vi "Update Digital Pattern Pattern Controls.vi"(8 "error in (no error)":errorcluster, 11 "Page Data in":T1={"SysExp Event"=refnum, "Init done"=FALSE, "Node Ptr"=18446744073709551615, "Ctrl Refs"={"Header"=refnum, "Pattern Plot"=refnum, "Zoom"=refnum, "Select Pattern"=refnum, "Add List"=refnum, "Remove List"=refnum, "Pattern Name"=refnum, "remove_add"=refnum, "remove_remove"=refnum, "add_remove"=refnum, "base_Length"=refnum, "base_teeth"=refnum, "base_Toothwidth"=refnum, "base_Offset"=refnum, "add_Tooth"=refnum, "add_Width"=refnum, "add_Offset"=refnum, "remove_Tooth"=refnum, "remove_Edge"=refnum, "Chart_Position"=refnum, "Chart_Tooth"=refnum, "Chart_Offset"=refnum, "add_add"=refnum, "pattern_remove"=refnum, "pattern_add"=refnum, "FPGA Resource"=refnum}, "SE ref"=refnum, "Patterns"=[], "Sel patterns"=[], "rotations"=0, "Need save"=FALSE, "Rem List"=0, "Add List"=0, "FPGA Resources"=[]} {"Node Ptr" format="%.0x"}) -> (0 "error out":errorcluster)   [LabVIEW 2017, in "Engine Simulation Toolkit System Explorer.lvlib"]
uses:
  Engine Simulation Toolkit System Explorer.lvlib
  Digital Patterns Page Data.ctl
  <vilib>/NI Veristand/Custom Device API/Custom Device Item Ref.ctl
  Digital Pattern.ctl
  Digital Pattern Base.ctl
  Digital Pattern Remove Edge.ctl
  Digital Pattern Add Pulse.ctl
  <vilib>/NI Veristand/Custom Device API/Custom Device API.lvlib
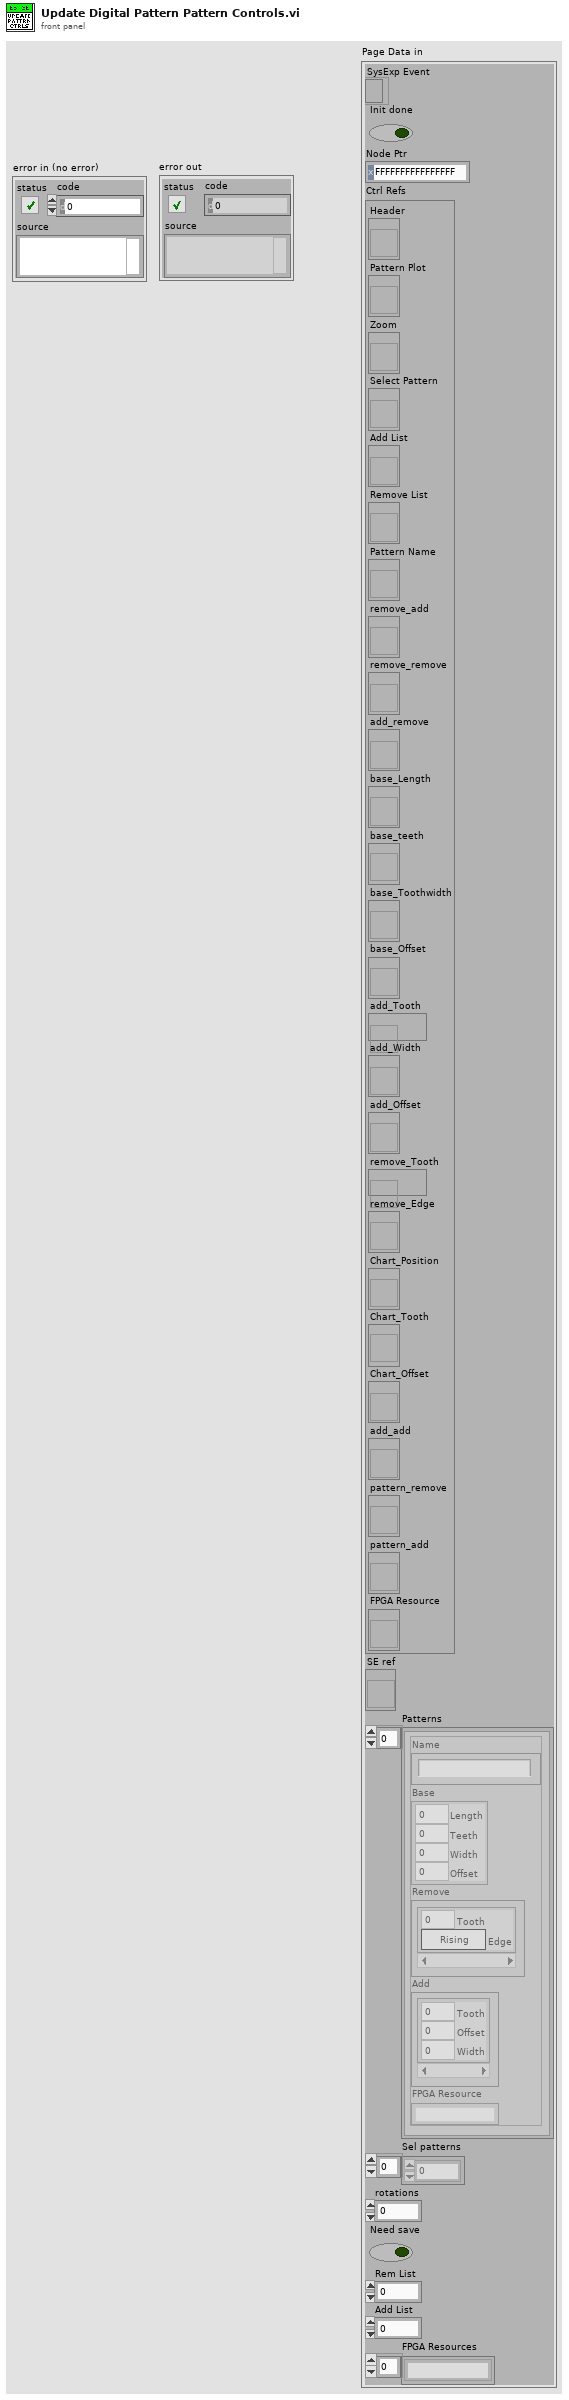
[diagram p1: front panel]
types:
  T1 = typedef "Engine Simulation Toolkit System Explorer.lvlib/Digital Patterns Page Data.ctl" = cluster{"SysExp Event":refnum<event-registration>, "Init done":bool, "Node Ptr":T2, "Ctrl Refs":cluster{"Header":refnum<vi>, "Pattern Plot":refnum<vi>, "Zoom":refnum<vi>, "Select Pattern":refnum<vi>, "Add List":refnum<vi>, "Remove List":refnum<vi>, "Pattern Name":refnum<vi>, "remove_add":refnum<vi>, "remove_remove":refnum<vi>, "add_remove":refnum<vi>, "base_Length":refnum<vi>, "base_teeth":refnum<vi>, "base_Toothwidth":refnum<vi>, "base_Offset":refnum<vi>, "add_Tooth":refnum<vi>, "add_Width":refnum<vi>, "add_Offset":refnum<vi>, "remove_Tooth":refnum<vi>, "remove_Edge":refnum<vi>, "Chart_Position":refnum<vi>, "Chart_Tooth":refnum<vi>, "Chart_Offset":refnum<vi>, "add_add":refnum<vi>, "pattern_remove":refnum<vi>, "pattern_add":refnum<vi>, "FPGA Resource":refnum<vi>}, "SE ref":refnum<vi>, "Patterns":T3[], "Sel patterns":i32[], "rotations":u16, "Need save":bool, "Rem List":i32, "Add List":i32, "FPGA Resources":string[]}
  T2 = typedef "Custom Device API.lvlib/Custom Device Item Ref.ctl" = u64
  T3 = typedef "Engine Simulation Toolkit System Explorer.lvlib/Digital Pattern.ctl" = cluster{"Name":string, "Base":T4, "Remove":T5[], "Add":T6[], "FPGA Resource":string}
  T4 = typedef "Engine Simulation Toolkit System Explorer.lvlib/Digital Pattern Base.ctl" = cluster{"Length":dbl, "Teeth":u16, "Width":dbl, "Offset":dbl}
  T5 = typedef "Engine Simulation Toolkit System Explorer.lvlib/Digital Pattern Remove Edge.ctl" = cluster{"Tooth":u16, "Edge":bool}
  T6 = typedef "Engine Simulation Toolkit System Explorer.lvlib/Digital Pattern Add Pulse.ctl" = cluster{"Tooth":u16, "Offset":dbl, "Width":dbl}
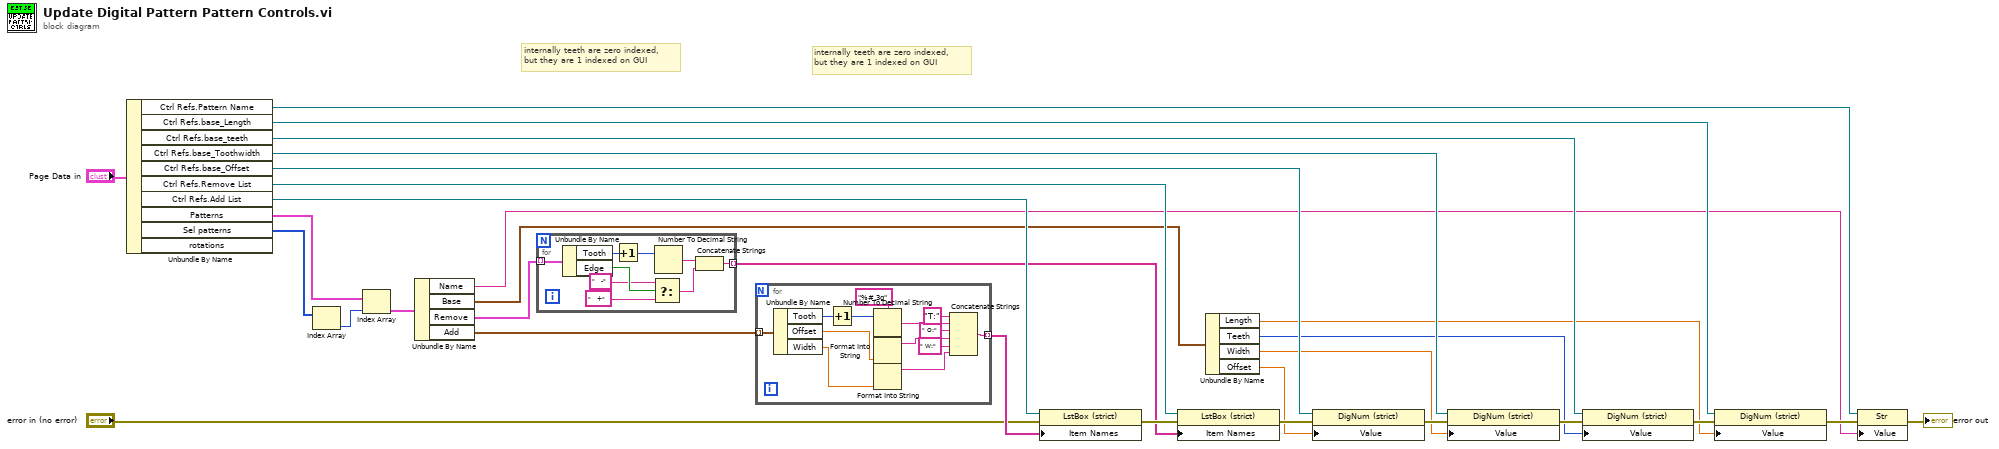
[diagram p0: block diagram]
diagram:
  # "internally teeth are zero indexed, but they are 1 indexed on GUI"
  # "internally teeth are zero indexed, but they are 1 indexed on GUI"
  n1 = Unbundle By Name("Page Data in") -> ("Ctrl Refs.Pattern Name"=w7:refnum<vi>, "Ctrl Refs.base_Length"=w10:refnum<vi>, "Ctrl Refs.base_teeth"=w12:refnum<vi>, "Ctrl Refs.base_Toothwidth"=w15:refnum<vi>, "Ctrl Refs.base_Offset"=w17:refnum<vi>, "Ctrl Refs.Remove List"=w20:refnum<vi>, "Ctrl Refs.Add List"=w24:refnum<vi>, "Patterns"=w2:T3[], "Sel patterns"=w29:i32[])  [unwired: 1 out]
  n2 = Index Array(array=w29) -> (element=w28:i32)  [unwired: 1 in]
  n3 = Index Array(array=w2, index=w28) -> (element=w27:T3)
  n4 = Unbundle By Name(w27) -> ("Name"=w6:string, "Base"=w19:T4, "Remove"=w23:T5[], "Add"=w26:T6[])
  n5 = for {
    tunnel: w23 -> [w39] mode=indexing
    tunnel: [w32] -> w21 mode=indexing
    n6 = Unbundle By Name(w39) -> ("Tooth"=w38:u16, "Edge"=w36:bool)
    n7 = Increment(x=w38) -> (x+1=w31:u16)
    n8 = Select(t="   -" ("string"), s=w36, f="   +" ("string")) -> (s? t:f=w35:string)
    n9 = Number To Decimal String(number=w31) -> (decimal integer string=w37:string)  [unwired: 1 in]
    n10 = Concatenate Strings(w37, w35) -> (w32:string)
  }
  n11 = for {
    tunnel: w26 -> [w52] mode=indexing
    tunnel: [w49] -> w25 mode=indexing
    w42 = "%#.3g" ("format string")
    n12 = Unbundle By Name(w52) -> ("Tooth"=w51:u16, "Offset"=w46:dbl, "Width"=w45:dbl)
    n13 = Increment(x=w51) -> (x+1=w40:u16)
    n14 = Number To Decimal String(number=w40) -> (decimal integer string=w50:string)  [unwired: 1 in]
    n15 = Format Into String(format string=w42, w46) -> (resulting string=w43:string)  [unwired: 2 in, 1 out]
    n16 = Format Into String(format string=w42, w45) -> (resulting string=w44:string)  [unwired: 2 in, 1 out]
    n17 = Concatenate Strings("T:" ("string"), w50, " O:" ("string"), w43, " W:" ("string"), w44) -> (w49:string)
  }
  n18 = property on="Property Node" class="LstBox (strict)"(reference=w24, error in="error in (no error)", "Item Names"=w25) -> (error out=w22:errorcluster)  [unwired: 1 out]
  n19 = property on="Property Node" class="LstBox (strict)"(reference=w20, error in=w22, "Item Names"=w21) -> (error out=w18:errorcluster)  [unwired: 1 out]
  n20 = Unbundle By Name(w19) -> ("Length"=w5:dbl, "Teeth"=w4:u16, "Width"=w14:dbl, "Offset"=w3:dbl)
  n21 = property on="Property Node" class="DigNum (strict)"(reference=w17, error in=w18, "Value"=w3) -> (error out=w16:errorcluster)  [unwired: 1 out]
  n22 = property on="Property Node" class="DigNum (strict)"(reference=w15, error in=w16, "Value"=w14) -> (error out=w13:errorcluster)  [unwired: 1 out]
  n23 = property on="Property Node" class="DigNum (strict)"(reference=w12, error in=w13, "Value"=w4) -> (error out=w11:errorcluster)  [unwired: 1 out]
  n24 = property on="Property Node" class="DigNum (strict)"(reference=w10, error in=w11, "Value"=w5) -> (error out=w8:errorcluster)  [unwired: 1 out]
  n25 = property on="Property Node" class="Str"(reference=w7, error in=w8, "Value"=w6) -> (error out=→"error out":errorcluster)  [unwired: 1 out]
